vi "Unit Test 2.vi"() -> ()   [LabVIEW 2018]
uses:
  PPLs/Oscilloscope/Parent/Oscilloscope.lvlibp/Custom Controls/Analog Channels.ctl
  PPLs/Oscilloscope/Parent/Oscilloscope.lvlibp/Custom Controls/Volts per Division.ctl
  PPLs/Oscilloscope/Parent/Oscilloscope.lvlibp/Custom Controls/Measurement.ctl
  PPLs/Oscilloscope/Parent/Oscilloscope.lvlibp/Custom Controls/Target Data.ctl
  PPLs/Oscilloscope/Parent/Oscilloscope.lvlibp/Custom Controls/Slope Edge.ctl
  PPLs/Oscilloscope/Parent/Oscilloscope.lvlibp/Custom Controls/Run Control.ctl
  PPLs/Oscilloscope/Parent/Oscilloscope.lvlibp/Custom Controls/Select Cursor.ctl
  PPLs/Oscilloscope/Parent/Oscilloscope.lvlibp/Custom Controls/Trigger Mode.ctl
  MSOX6004.lvclass
  PPLs/Oscilloscope/Parent/Oscilloscope.lvlibp/Oscilloscope.lvclass
  PPLs/Oscilloscope/Parent/Oscilloscope.lvlibp
  C:/Projects/LabVIEW/PPLs/Oscilloscope/Parent/Oscilloscope.lvlibp/Oscilloscope.lvclass
panel:
  in  "Trigger Mode":T1
  out "Triggered?":bool
  out "Statistics 2":T2
  in  "Multiple Stats":T5
  out "Multiple Statistics":T6(array[cluster])
  out "Command Rsp":string
  in  "Command":string
  out "Status Array":bool[](array[boolean])
  out "Position":dbl format="%.9f"
  in  "Cursor":T7
  in  "Channel Label":cluster{"Analog Channels":T3, "Label":string}
  in  "Run Control Start":T8
  in  "Signals Delay Measurement":T10
  out "Delay":dbl
  in  "Statistics Measurement":T11={"Channels"=enum."1", "Measurement"=enum."Rise Time", "No. Reads"=2000}
  out "Statistics":T2
  in  "Div. Delay":dbl format="%#_6e"
  in  "Single Measurement":T13
  out "Measurement":dbl
  out "Waveforms":waveform(dbl)[](graph)
  in  "Intensity (1-100)":i8=100 min=1 max=100 step=1
  in  "Edge Trigger":T14 {"Trigger Slope (0: Rising)" items=["Rising", "Falling", "Either"]}
  in  "Vertical Offset":cluster{"Channels":T3, "Offset":dbl}[](array[cluster]) {"Offset" format="%#_13g"}
  in  "Secs/div":dbl
  in  "V/div":T15
  in  "Active Channel(s)":T3[](array[typedef])
  out "error out":errorcluster
  in  "Commands":T16(array[ring])
  in  "Resource":refnum<visa-resource-name>="TCPIP0::192.168.0.50::INSTR"
  # "do it after RUN and before\nstarting stats"
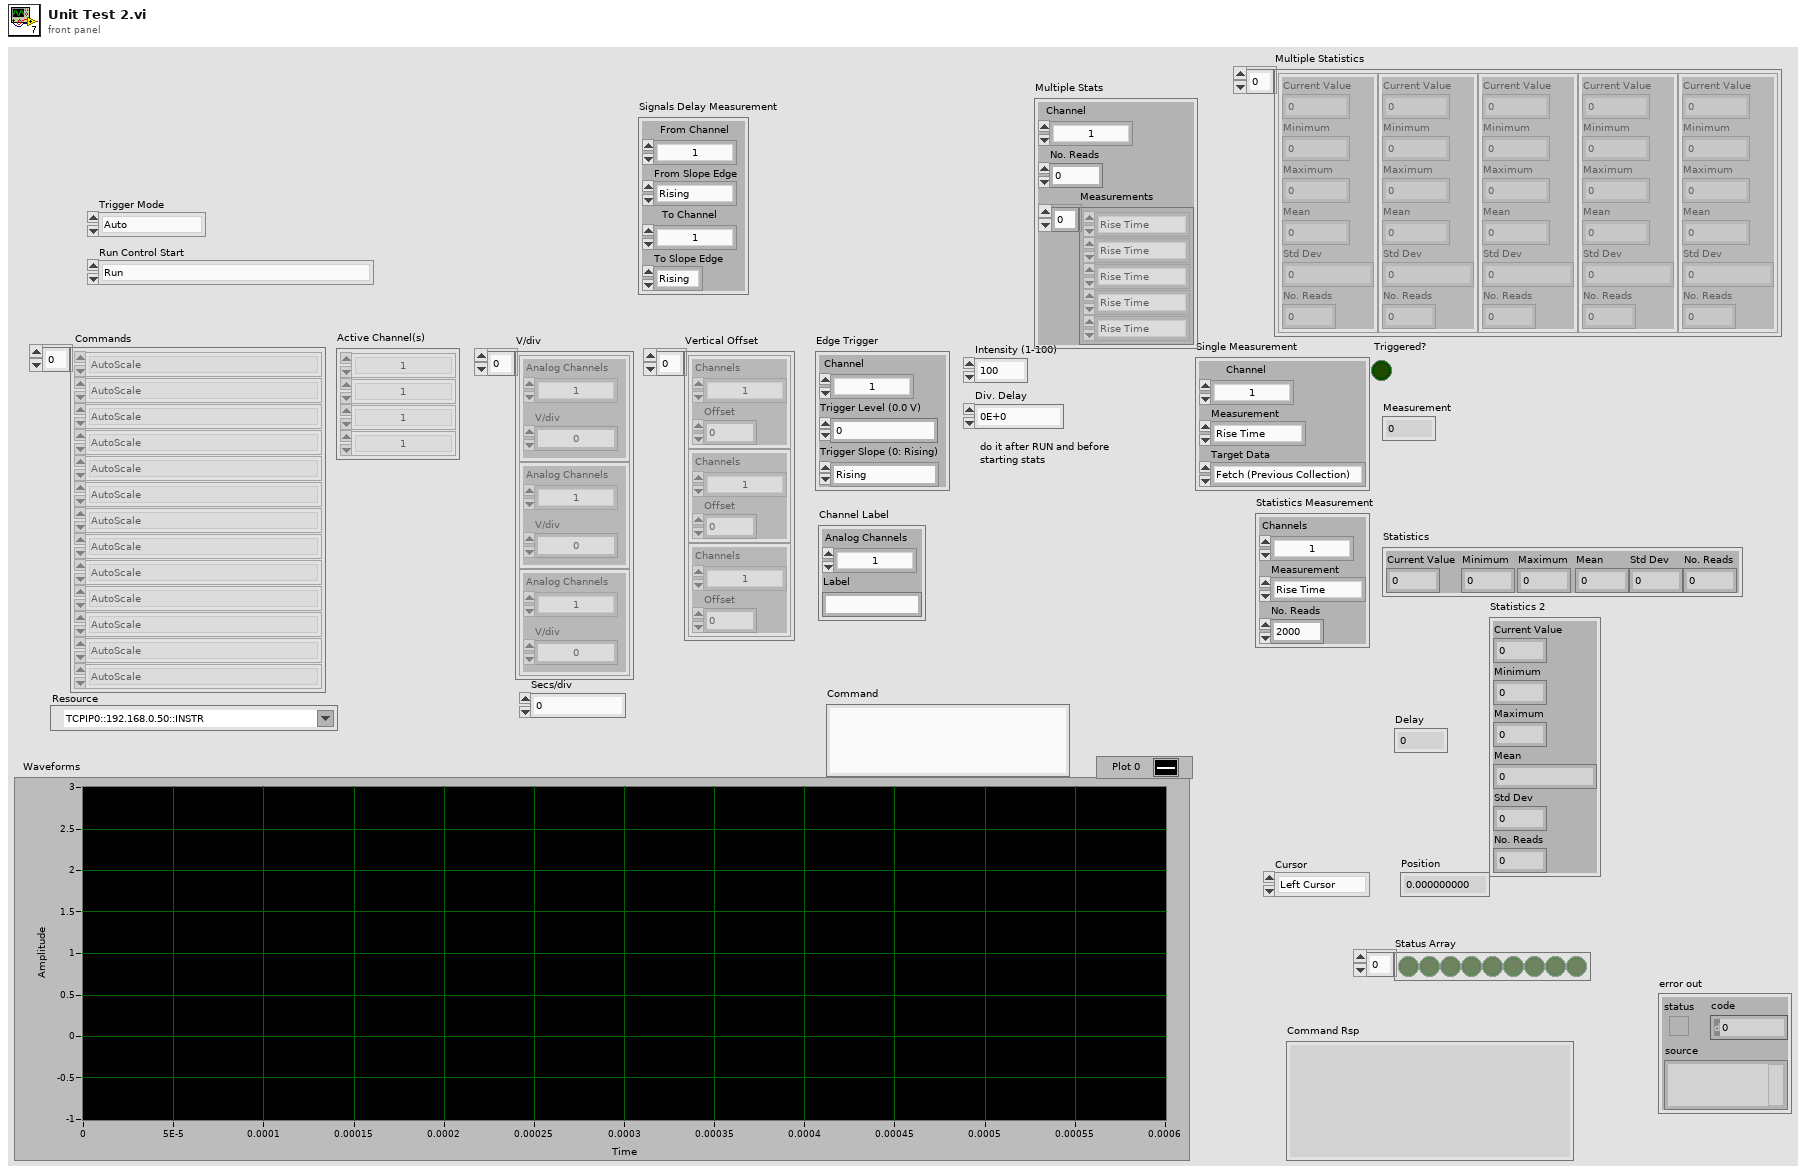
[diagram p1: front panel]
types:
  T1 = typedef "Oscilloscope.lvlibp/Trigger Mode.ctl" = enum16{"Auto", "Normal"}
  T2 = cluster{"Current Value":dbl, "Minimum":dbl, "Maximum":dbl, "Mean":dbl, "Std Dev":dbl, "No. Reads":dbl}
  T3 = typedef "Oscilloscope.lvlibp/Analog Channels.ctl" = enum16{"1", "2", "3", "4", "5", "6", "7", "8", "9", "10", "11", "12", "13", "14", "15", "16"}
  T4 = typedef "Oscilloscope.lvlibp/Measurement.ctl" = enum16{"Rise Time", "Fall Time", "Frequency", "Period", "RMS (V)", "Peak-Peak (V)", "Max (V)", "Min (V)", "High State (V)", "Low State (V)", "Average (V)", "Width (Negative)", "Width (Positive)", "Duty Cycle (Negative)", "Duty Cycle (Positive)", "Amplitude", "Cycle RMS (V)", "Cycle Avg (V)", "Overshoot", "Preshoot", "Time at Max", "Frequency Counter", "Time at Min", "Delay", "Value at Time", "Phase", "Time at Value", "Time of Edge", "Area", "Burst Width", "Falling Edge Count", "Rising Edge Count", "Falling Pulse Count", "Rising Pulse Count", "Std Dev", "Pulse Width"}
  T5 = cluster{"Channel":T3, "No. Reads":i32, "Measurements":T4[]}
  T6 = cluster{"Current Value":dbl, "Minimum":dbl, "Maximum":dbl, "Mean":dbl, "Std Dev":dbl, "No. Reads":dbl}[]
  T7 = typedef "Oscilloscope.lvlibp/Select Cursor.ctl" = enum16{"Left Cursor", "Right Cursor", "Top Cursor", "Bottom Cursor"}
  T8 = typedef "Oscilloscope.lvlibp/Run Control.ctl" = enum16{"Run", "Single", "Stop"}
  T9 = typedef "Oscilloscope.lvlibp/Slope Edge.ctl" = enum16{"Rising", "Falling"}
  T10 = cluster{"From Channel":T3, "From Slope Edge":T9, "To Channel":T3, "To Slope Edge":T9}
  T11 = cluster{"Channels":T3, "Measurement":T4, "No. Reads":i32}
  T12 = typedef "Oscilloscope.lvlibp/Target Data.ctl" = enum16{"Fetch (Previous Collection)", "Measure (New Collection)"}
  T13 = cluster{"Channel":T3, "Measurement":T4, "Target Data":T12}
  T14 = cluster{"Channel":T3, "Trigger Level (0.0 V)":dbl, "Trigger Slope (0: Rising)":u16}
  T15 = typedef "Oscilloscope.lvlibp/Volts per Division.ctl" = cluster{"Analog Channels":T3, "V/div":dbl}[]
  T16 = enum16{"AutoScale", "Lock Panel", "Take Screenshot", "Select Active Channels", "Manual Scale", "Vertical Offset", "Set Edge Trigger", "Waveform Intensity", "Read Waveform(s)", "Measure Waveform", "Set Horizontal Delay", "Read Statistics", "Measure Signals Delay", "Run Control", "Set Channel Label", "Read Cursors", "Status", "Send Command", "Read Multiple Stats", "verify Trigger State", "Set Trigger Mode", "End"}[]
  T17 = enum16{"AutoScale", "Lock Panel", "Take Screenshot", "Select Active Channels", "Manual Scale", "Vertical Offset", "Set Edge Trigger", "Waveform Intensity", "Read Waveform(s)", "Measure Waveform", "Set Horizontal Delay", "Read Statistics", "Measure Signals Delay", "Run Control", "Set Channel Label", "Read Cursors", "Status", "Send Command", "Read Multiple Stats", "verify Trigger State", "Set Trigger Mode", "End"}
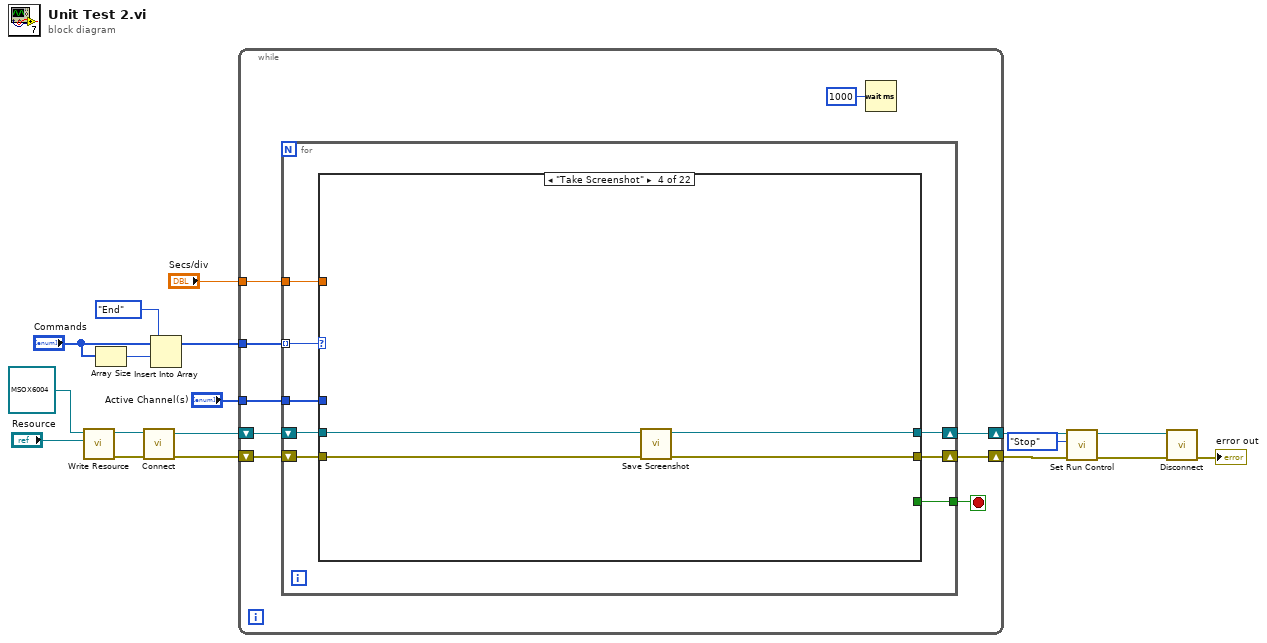
[diagram p0: block diagram]
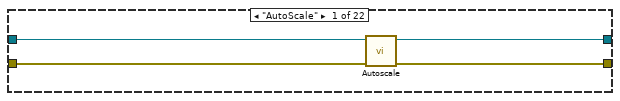
[diagram p2: hidden frame]
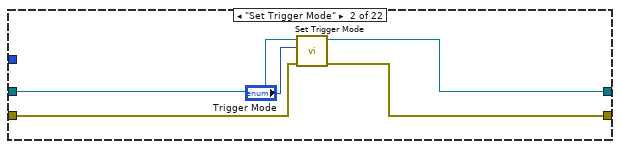
[diagram p3: hidden frame]
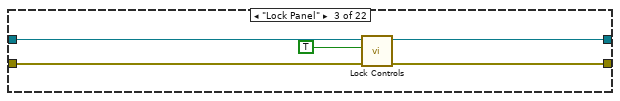
[diagram p4: hidden frame]
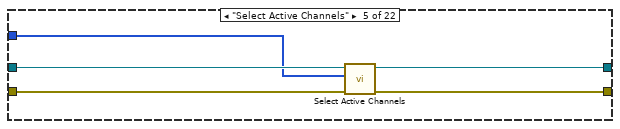
[diagram p5: hidden frame]
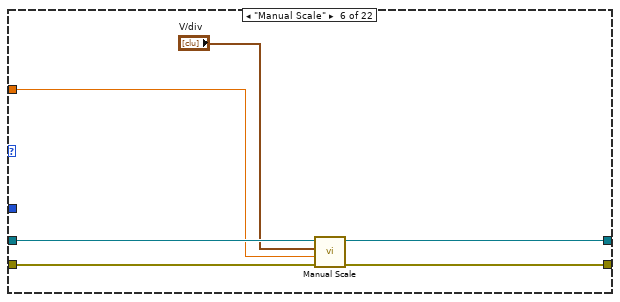
[diagram p6: hidden frame]
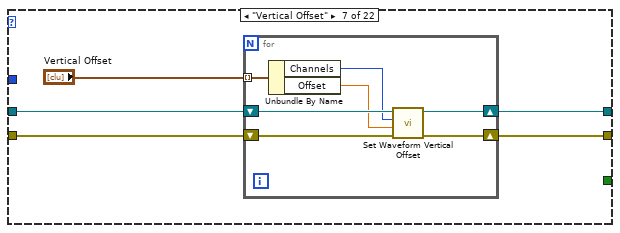
[diagram p7: hidden frame]
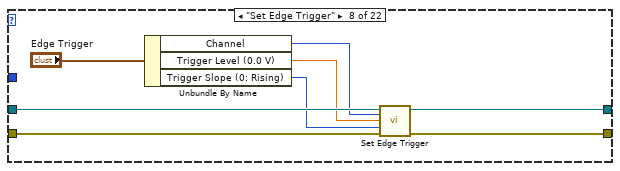
[diagram p8: hidden frame]
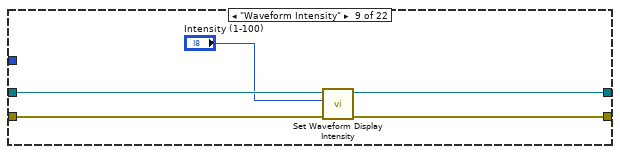
[diagram p9: hidden frame]
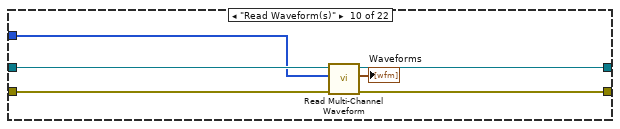
[diagram p10: hidden frame]
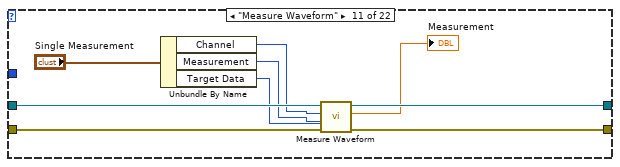
[diagram p11: hidden frame]
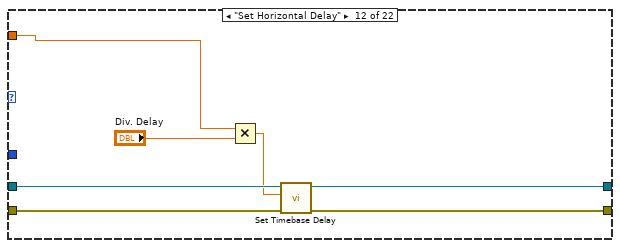
[diagram p12: hidden frame]
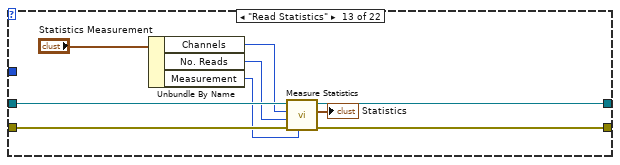
[diagram p13: hidden frame]
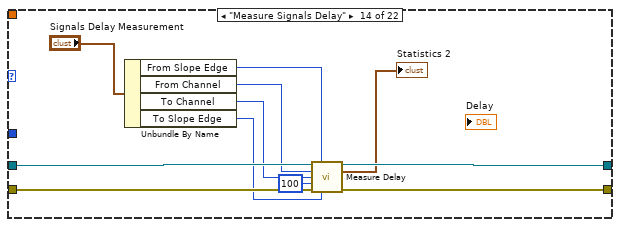
[diagram p14: hidden frame]
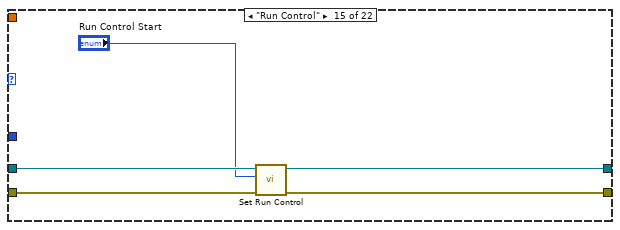
[diagram p15: hidden frame]
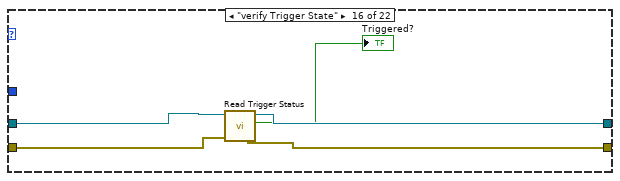
[diagram p16: hidden frame]
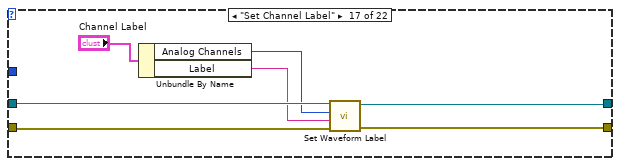
[diagram p17: hidden frame]
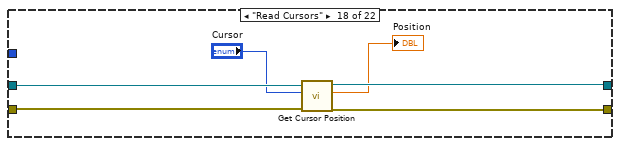
[diagram p18: hidden frame]
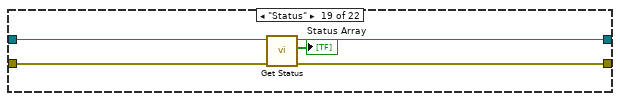
[diagram p19: hidden frame]
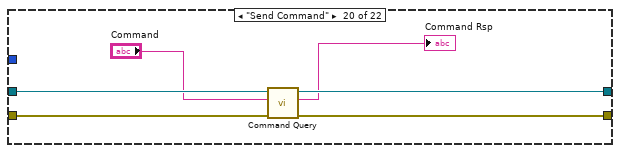
[diagram p20: hidden frame]
diagram:
  n1 = call "Write Resource.vi"("Resource"="Resource", "Oscilloscope in"=refnum<class "MSOX6004.lvclass"> refnum ("MSOX6004.lvlib:MSOX6004.lvclass")) -> ("error out"=w17:errorcluster, "Oscilloscope out"=w18:refnum<class "MSOX6004.lvclass">)  [unwired: 8 in]
  n2 = Array Size(array="Commands") -> (size(s)=w11:i32)
  n3 = call-dynamic "Connect.vi"("error in (no error)"=w17, "MSOX6004 in"=w18) -> ("error out"=w15:errorcluster, "MSOX6004 out"=w16:refnum<class "MSOX6004.lvclass">)  [unwired: 8 in]
  n4 = Insert Into Array(array="Commands", index=w11, new element=T17."End" ("new element/subarray")) -> (w9:T16)
  n5 = while {
    tunnel: w9 -> [w25]
    shift-right: [w24] -> w5
    shift-left: w16 -> [w27]
    shift-right: [w23] -> w3
    shift-left: w15 -> [w26]
    tunnel: "Active Channel(s)" -> [w22]
    tunnel: "Secs/div" -> [w21]
    stop <- w20 stop-if-true
    n6 = for {
      tunnel: w25 -> [w33] mode=indexing
      shift-right: [w32] -> w24
      shift-left: w27 -> [w35]
      shift-right: [w31] -> w23
      shift-left: w26 -> [w34]
      tunnel: w22 -> [w30]
      tunnel: w21 -> [w29]
      tunnel: [w28] -> w20
      n7 = case shown="\"Take Screenshot\"" w33 {
        tunnel: w35 -> [w39 w44 w49 w53 w57 w61 w69 w84 w88 w95 w102 w110 w120 w131 w136 w141 w148 w154 w159 w165 w174 w177]
        tunnel: w34 -> [w38 w43 w48 w52 w58 w64 w68 w83 w89 w94 w104 w111 w117 w129 w135 w140 w147 w153 w158 w164 w172 w176]
        tunnel: [w37 w42 w47 w51 w56 w62 w67 w82 w87 w93 w101 w109 w119 w130 w134 w139 w146 w152 w157 w163 w173 w177] -> w32
        tunnel: [w36 w41 w46 w50 w55 w63 w66 w81 w86 w92 w103 w108 w118 w128 w133 w138 w145 w151 w156 w162 w171 w176] -> w31
        tunnel: w30 -> [_ _ _ _ w54 _ _ _ _ w91 _ _ _ _ _ _ _ _ _ _ _ _]
        tunnel: w29 -> [_ _ _ _ _ w59 _ _ _ _ _ w105 _ _ _ _ _ _ _ _ _ _]
        tunnel: [_ _ _ _ _ _ _ _ _ _ _ _ _ _ _ _ _ _ _ _ _ TRUE] -> w28
        frame "AutoScale" {
          n8 = call-dynamic "Autoscale.vi"("error in (no error)"=w38, "MSOX6004 in"=w39) -> ("error out"=w36:errorcluster, "MSOX6004 out"=w37:refnum<class "MSOX6004.lvclass">)  [unwired: 8 in]
        }
        frame "Set Trigger Mode" {
          n9 = call-dynamic "Set Trigger Mode.vi"("error in (no error)"=w43, "Trigger Mode"="Trigger Mode", "MSOX6004 in"=w44) -> ("error out"=w41:errorcluster, "MSOX6004 out"=w42:refnum<class "MSOX6004.lvclass">)  [unwired: 7 in]
        }
        frame "Lock Panel" {
          n10 = call-dynamic "Lock Controls.vi"("error in (no error)"=w48, "Lock Controls?"=TRUE, "MSOX6004 in"=w49) -> ("error out"=w46:errorcluster, "MSOX6004 out"=w47:refnum<class "MSOX6004.lvclass">)  [unwired: 7 in]
        }
        frame "Take Screenshot" {
          n11 = call-dynamic "Save Screenshot.vi"("error in (no error)"=w52, "MSOX6004 in"=w53) -> ("error out"=w50:errorcluster, "MSOX6004 out"=w51:refnum<class "MSOX6004.lvclass">)  [unwired: 8 in]
        }
        frame "Select Active Channels" {
          n12 = call-dynamic "Select Active Channels.vi"("error in (no error)"=w58, "Active Channel(s)"=w54, "MSOX6004 in"=w57) -> ("error out"=w55:errorcluster, "MSOX6004 out"=w56:refnum<class "MSOX6004.lvclass">)  [unwired: 7 in]
        }
        frame "Manual Scale" {
          n13 = call-dynamic "Manual Scale.vi"("error in (no error)"=w64, "Secs/div"=w59, "V/div"="V/div", "MSOX6004 in"=w61) -> ("error out"=w63:errorcluster, "MSOX6004 out"=w62:refnum<class "MSOX6004.lvclass">)  [unwired: 6 in]
        }
        frame "Vertical Offset" {
          n14 = for {
            shift-right: [w74] -> w67
            shift-left: w69 -> [w76]
            shift-right: [w73] -> w66
            shift-left: w68 -> [w75]
            tunnel: "Vertical Offset" -> [w72] mode=indexing
            n15 = Unbundle By Name(w72) -> ("Channels"=w71:T3, "Offset"=w70:dbl)
            n16 = call-dynamic "Set Waveform Vertical Offset.vi"("error in (no error)"=w75, "Offset Divisions"=w70, "Analog Channels"=w71, "MSOX6004 in"=w76) -> ("error out"=w73:errorcluster, "MSOX6004 out"=w74:refnum<class "MSOX6004.lvclass">)  [unwired: 6 in]
          }
        }
        frame "Set Edge Trigger" {
          n17 = Unbundle By Name("Edge Trigger") -> ("Channel"=w79:T3, "Trigger Level (0.0 V)"=w78:dbl, "Trigger Slope (0: Rising)"=w77:u16)
          n18 = call-dynamic "Set Edge Trigger.vi"("Trigger Slope (0: Rising)"=w77, "error in (no error)"=w83, "Trigger Level (0.0 V)"=w78, "Analog Channel"=w79, "MSOX6004 in"=w84) -> ("error out"=w81:errorcluster, "MSOX6004 out"=w82:refnum<class "MSOX6004.lvclass">)  [unwired: 5 in]
        }
        frame "Waveform Intensity" {
          n19 = call-dynamic "Set Waveform Display Intensity.vi"("error in (no error)"=w89, "Intensity (1-100)"="Intensity (1-100)", "MSOX6004 in"=w88) -> ("error out"=w86:errorcluster, "MSOX6004 out"=w87:refnum<class "MSOX6004.lvclass">)  [unwired: 7 in]
        }
        frame "Read Waveform(s)" {
          n20 = call-dynamic "Read Multi-Channel Waveform.vi"("error in (no error)"=w94, "Channels"=w91, "MSOX6004 in"=w95) -> ("error out"=w92:errorcluster, "Waveform"=→"Waveforms":waveform(dbl)[], "MSOX6004 out"=w93:refnum<class "MSOX6004.lvclass">)  [unwired: 6 in]
        }
        frame "Measure Waveform" {
          n21 = Unbundle By Name("Single Measurement") -> ("Channel"=w98:T3, "Measurement"=w97:T4, "Target Data"=w96:T12)
          n22 = call-dynamic "Measure Waveform.vi"("Target Data"=w96, "error in (no error)"=w104, "Measurement"=w97, "Channel"=w98, "MSOX6004 in"=w102) -> ("error out"=w103:errorcluster, "Measurement"=→"Measurement":dbl, "MSOX6004 out"=w101:refnum<class "MSOX6004.lvclass">)  [unwired: 4 in]
        }
        frame "Set Horizontal Delay" {
          n23 = Multiply(x=w105, y="Div. Delay") -> (x*y=w106:dbl)
          n24 = call-dynamic "Set Timebase Delay.vi"("error in (no error)"=w111, "Delay"=w106, "MSOX6004 in"=w110) -> ("error out"=w108:errorcluster, "MSOX6004 out"=w109:refnum<class "MSOX6004.lvclass">)  [unwired: 7 in]
        }
        frame "Read Statistics" {
          n25 = Unbundle By Name("Statistics Measurement") -> ("Channels"=w114:T3, "No. Reads"=w113:i32, "Measurement"=w112:T4)
          n26 = call-dynamic "Measure Statistics.vi"("Measurement"=w112, "error in (no error)"=w117, "No. Reads"=w113, "Channel"=w114, "MSOX6004 in"=w120) -> ("error out"=w118:errorcluster, "Statistics"=→"Statistics":T2, "MSOX6004 out"=w119:refnum<class "MSOX6004.lvclass">)  [unwired: 4 in]
        }
        frame "Measure Signals Delay" {
          n27 = Unbundle By Name("Signals Delay Measurement") -> ("From Slope Edge"=w125:T9, "From Channel"=w126:T3, "To Channel"=w124:T3, "To Slope Edge"=w123:T9)
          n28 = call-dynamic "Measure Delay.vi"("MSOX6004 in"=w131, "From Slope Edge"=w125, "From Channel"=w126, "To Channel"=w124, "No. Reads"=100, "error in (no error)"=w129, "To Slope Edge"=w123) -> ("MSOX6004 out"=w130:refnum<class "MSOX6004.lvclass">, "Statistics"=→"Statistics 2":T2, "error out"=w128:errorcluster)  [unwired: 6 in]
        }
        frame "Run Control" {
          n29 = call-dynamic "Set Run Control.vi"("error in (no error)"=w135, "Run Control"="Run Control Start", "MSOX6004 in"=w136) -> ("error out"=w133:errorcluster, "MSOX6004 out"=w134:refnum<class "MSOX6004.lvclass">)  [unwired: 7 in]
        }
        frame "verify Trigger State" {
          n30 = call-dynamic "Read Trigger Status.vi"("error in (no error)"=w140, "MSOX6004 in"=w141) -> ("error out"=w138:errorcluster, "Triggered?"=→"Triggered?":bool, "MSOX6004 out"=w139:refnum<class "MSOX6004.lvclass">)  [unwired: 7 in]
        }
        frame "Set Channel Label" {
          n31 = Unbundle By Name("Channel Label") -> ("Analog Channels"=w143:T3, "Label"=w142:string)
          n32 = call-dynamic "Set Waveform Label.vi"("error in (no error)"=w147, "Label"=w142, "Analog Channels"=w143, "MSOX6004 in"=w148) -> ("error out"=w145:errorcluster, "MSOX6004 out"=w146:refnum<class "MSOX6004.lvclass">)  [unwired: 6 in]
        }
        frame "Read Cursors" {
          n33 = call-dynamic "Get Cursor Position.vi"("error in (no error)"=w153, "Cursor"="Cursor", "MSOX6004 in"=w154) -> ("error out"=w151:errorcluster, "Position"=→"Position":dbl, "MSOX6004 out"=w152:refnum<class "MSOX6004.lvclass">)  [unwired: 6 in]
        }
        frame "Status" {
          n34 = call-dynamic "Get Status.vi"("error in (no error)"=w158, "MSOX6004 in"=w159) -> ("error out"=w156:errorcluster, "Status Array"=→"Status Array":bool[], "MSOX6004 out"=w157:refnum<class "MSOX6004.lvclass">)  [unwired: 7 in]
        }
        frame "Send Command" {
          n35 = call "Command Query.vi"("error in (no error)"=w164, "Command"="Command", "MSOX6004 in"=w165) -> ("error out"=w162:errorcluster, "Response"=→"Command Rsp":string, "MSOX6004 out"=w163:refnum<class "MSOX6004.lvclass">)  [unwired: 6 in]
        }
        frame "Read Multiple Stats" {
          n36 = Unbundle By Name("Multiple Stats") -> ("Channel"=w168:T3, "No. Reads"=w167:i32, "Measurements"=w166:T4[])
          n37 = call-dynamic "Measure Statistics (Multiple).vi"("Measurements"=w166, "error in (no error)"=w172, "No. Reads"=w167, "Channel"=w168, "MSOX6004 in"=w174) -> ("error out"=w171:errorcluster, "Multiple Statistics"=→"Multiple Statistics":T6, "MSOX6004 out"=w173:refnum<class "MSOX6004.lvclass">)  [unwired: 4 in]
        }
        frame "End" {
        }
      }
    }
    n38 = Wait (ms)(milliseconds to wait=u32 1000) -> ()  [unwired: 1 out]
  }
  n39 = call-dynamic "Set Run Control.vi"("error in (no error)"=w3, "Run Control"=Run_Control."Stop", "MSOX6004 in"=w5) -> ("error out"=w2:errorcluster, "MSOX6004 out"=w4:refnum<class "MSOX6004.lvclass">)  [unwired: 7 in]
  n40 = call-dynamic "Disconnect.vi"("error in (no error)"=w2, "MSOX6004 in"=w4) -> ("error out"=→"error out":errorcluster)  [unwired: 8 in, 1 out]
